vi "Init.vi"(8 "error in":errorcluster, 11 "Messaging Buffer in":refnum<class "Message Buffer.lvclass">) -> (0 "error out":errorcluster, 3 "Messaging Buffer out":refnum<class "Message Buffer.lvclass">)   [LabVIEW 2024, in "PCAN.lvlib" / "Message Buffer.lvclass"]
uses:
  Message Buffer.lvclass
  Message Buffer.lvclass/Message Buffer.ctl
  CAN Message/CAN Message.lvclass
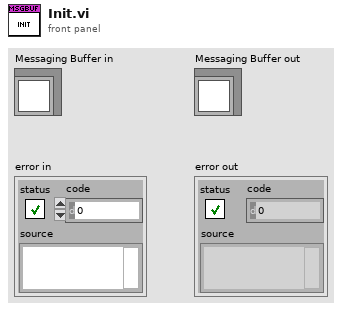
[diagram p1: front panel]
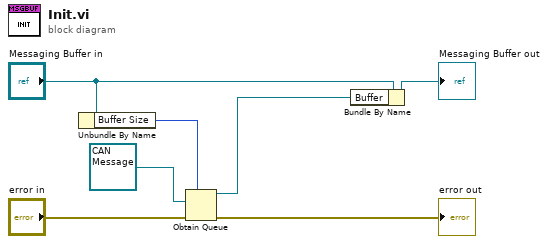
[diagram p0: block diagram]
diagram:
  n1 = Unbundle By Name("Messaging Buffer in") -> ("Buffer Size"=w2:u32)
  n2 = Obtain Queue(max queue size (-1, unlimited)=w2, element data type=refnum<class "CAN Message.lvclass"> refnum ("PCAN.lvlib:CAN Message"), error in (no error)="error in") -> (queue out=w1:refnum<queue>, error out=→"error out":errorcluster)  [unwired: 2 in, 1 out]
  n3 = Bundle By Name(cluster="Messaging Buffer in", "Buffer"=w1) -> (→"Messaging Buffer out":refnum<class "Message Buffer.lvclass">)
